vi "lockin_controller.vi"(10 "Numerical Argument":dbl, 11 "Command":T1(ring)=enum."Get Amplitude") -> (3 "Response":string)   [LabVIEW 2021]
panel:
  # "LOCKIN AMPLIFIER CONTROLLER"
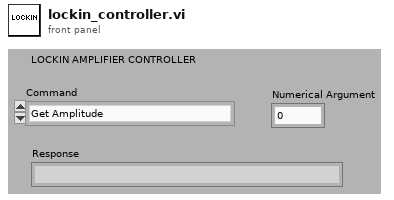
[diagram p1: front panel]
types:
  T1 = enum16{"Set Amplitude", "Get Amplitude", "Set Frequency", "Get Frequency", "Set Harmonic", "Get Harmonic", "Set Phase", "Get Phase", "Auto Phase", "Add to Phase", "Autogain", "Set Time Constant", "Get Time Constant", "Set Sensitivity", "Get Sensitivity", "Set Input A", "Set Input A-B", "Get Input Setting", "Set Offset", "Get Offset"}
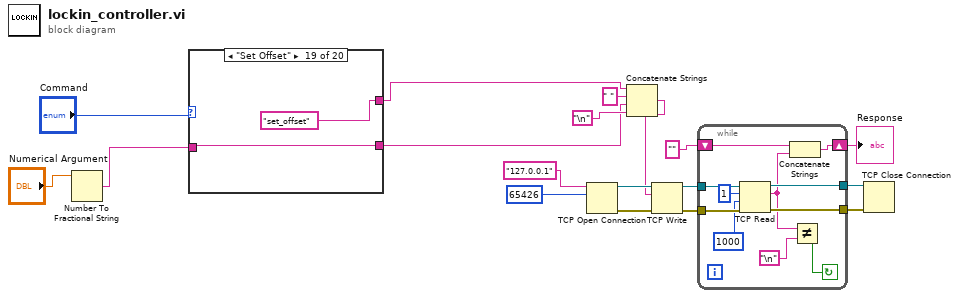
[diagram p0: block diagram]
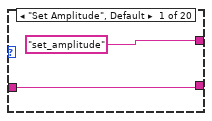
[diagram p2: hidden frame]
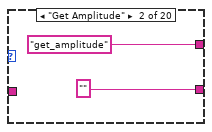
[diagram p3: hidden frame]
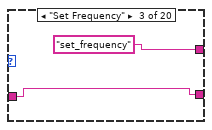
[diagram p4: hidden frame]
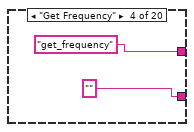
[diagram p5: hidden frame]
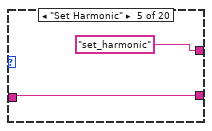
[diagram p6: hidden frame]
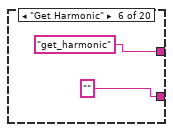
[diagram p7: hidden frame]
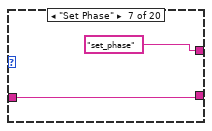
[diagram p8: hidden frame]
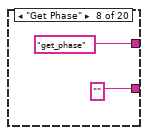
[diagram p9: hidden frame]
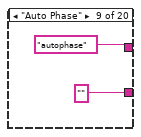
[diagram p10: hidden frame]
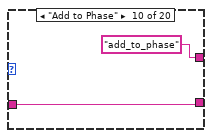
[diagram p11: hidden frame]
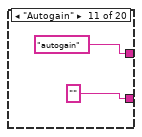
[diagram p12: hidden frame]
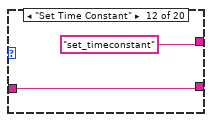
[diagram p13: hidden frame]
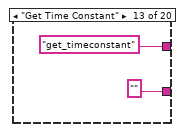
[diagram p14: hidden frame]
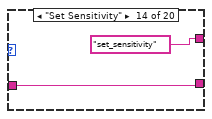
[diagram p15: hidden frame]
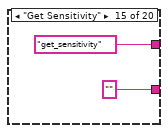
[diagram p16: hidden frame]
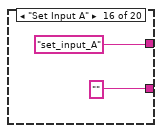
[diagram p17: hidden frame]
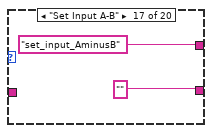
[diagram p18: hidden frame]
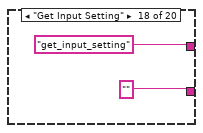
[diagram p19: hidden frame]
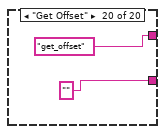
[diagram p20: hidden frame]
diagram:
  n1 = Number To Fractional String(number="Numerical Argument") -> (F-format string=w3:string)  [unwired: 3 in]
  n2 = case shown="\"Set Offset\"" "Command" {
    tunnel: ["set_amplitude" ("data in") "get_amplitude" ("data in") "set_frequency" ("data in") "get_frequency" ("data in") "set_harmonic" ("data in") "get_harmonic" ("data in") "set_phase" ("data in") "get_phase" ("data in") "autophase" ("data in") "add_to_phase" ("data in") "autogain" ("data in") "set_timeconstant" ("data in") "get_timeconstant" ("data in") "set_sensitivity" ("data in") "get_sensitivity" ("data in") "set_input_A" ("data in") "set_input_AminusB" ("data in") "get_input_setting" ("data in") "set_offset" ("data in") "get_offset" ("data in")] -> w1
    tunnel: [w19 "" ("string") w23 "" ("string") w27 "" ("string") w31 "" ("string") "" ("string") w37 "" ("string") w42 "" ("string") w45 "" ("string") "" ("string") "" ("string") "" ("string") w55 "" ("string")] -> w4
    tunnel: w3 -> [w19 _ w23 _ w27 _ w31 _ _ w37 _ w42 _ w45 _ _ _ _ w55 _]
    frame "Set Amplitude", Default {
    }
    frame "Get Amplitude" {
    }
    frame "Set Frequency" {
    }
    frame "Get Frequency" {
    }
    frame "Set Harmonic" {
    }
    frame "Get Harmonic" {
    }
    frame "Set Phase" {
    }
    frame "Get Phase" {
    }
    frame "Auto Phase" {
    }
    frame "Add to Phase" {
    }
    frame "Autogain" {
    }
    frame "Set Time Constant" {
    }
    frame "Get Time Constant" {
    }
    frame "Set Sensitivity" {
    }
    frame "Get Sensitivity" {
    }
    frame "Set Input A" {
    }
    frame "Set Input A-B" {
    }
    frame "Get Input Setting" {
    }
    frame "Set Offset" {
    }
    frame "Get Offset" {
    }
  }
  n3 = TCP Open Connection(address="127.0.0.1", remote port or service name=u16 65426) -> (connection ID=w16:refnum<k5>, error out=w15:errorcluster)  [unwired: 3 in]
  n4 = Concatenate Strings(w1, " " ("string"), w4, "\n") -> (w8:string)
  n5 = TCP Write(connection ID=w16, data in=w8, error in (no error)=w15) -> (connection ID out=w13:refnum<k5>, error out=w14:errorcluster)  [unwired: 1 in, 1 out]
  n6 = while {
    tunnel: w14 -> [w69]
    tunnel: w13 -> [w68]
    tunnel: [w67] -> w12
    tunnel: [w66] -> w11
    shift-right: [w62] -> w9
    shift-left: "" ("string") -> [w63]
    stop <- w61 continue-if-true
    n7 = TCP Read(connection ID=w68, bytes to read=1, error in (no error)=w69, 9:1000 ("timeout ms (25000)")) -> (connection ID out=w66:refnum<k5>, data out=w60:string, error out=w67:errorcluster)  [unwired: 1 in]
    n8 = Concatenate Strings(w63, w60) -> (w62:string)
    n9 = Not Equal?(x=w60, y="\n") -> (x != y?=w61:bool)
  }
  "Response" <- w9
  n10 = TCP Close Connection(connection ID=w11, error in (no error)=w12) -> ()  [unwired: 1 in, 2 out]
